vi "Icon Templates.vi"() -> ()   [LabVIEW 2013]
panel:
  out "Ring":u16(ring)
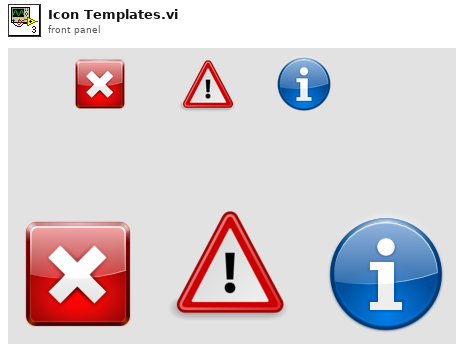
[diagram p1: front panel]
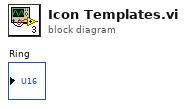
[diagram p0: block diagram]
diagram:
